vi "HW.vi"() -> ()   [LabVIEW 2018]
panel:
  out "String":string
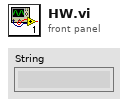
[diagram p1: front panel]
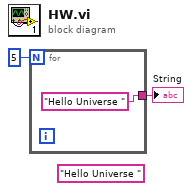
[diagram p0: block diagram]
diagram:
  (unwired) "Hello Universe "
  n1 = for {
    N: 5 -> [_]
    tunnel: ["Hello Universe "] -> w1
  }
  "String" <- w1
